vi "AuthAtServer.vi"(8 "password":string, 9 "login":string, 10 "Port":u32, 11 "Adress":string) -> (0 "MulticastAdress":string, 1 "AuthKey":string, 3 "error out":errorcluster)   [LabVIEW 2016]
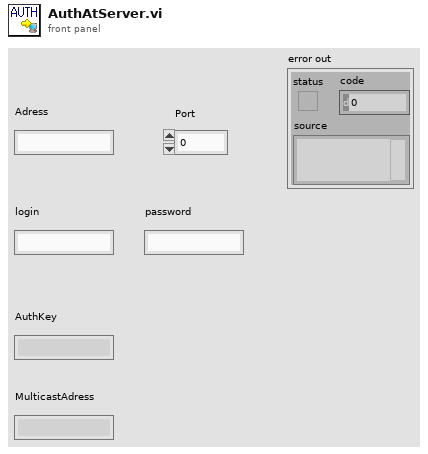
[diagram p1: front panel]
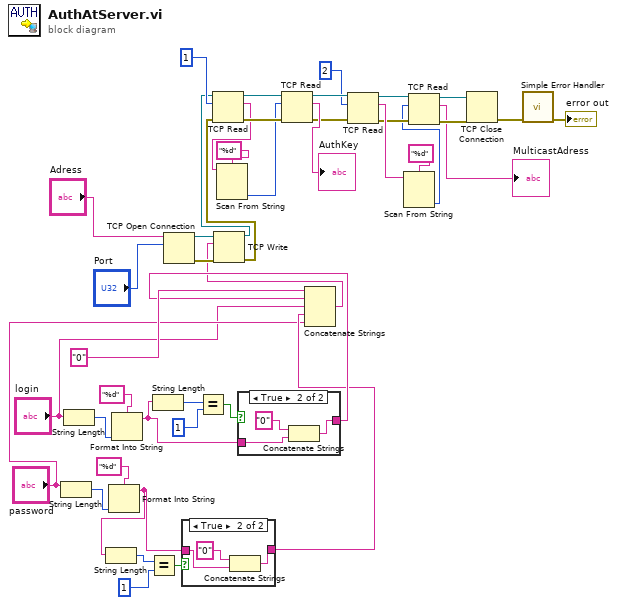
[diagram p0: block diagram]
diagram:
  n1 = String Length(string="password") -> (length=w39:i32)
  n2 = String Length(string="login") -> (length=w41:i32)
  n3 = Format Into String(format string="%d", w39) -> (resulting string=w32:string)  [unwired: 2 in, 1 out]
  n4 = String Length(string=w32) -> (length=w35:i32)
  n5 = Format Into String(format string="%d", w41) -> (resulting string=w28:string)  [unwired: 2 in, 1 out]
  n6 = Equal?(x=w35, y=1) -> (x = y?=w33:bool)
  n7 = String Length(string=w28) -> (length=w31:i32)
  n8 = TCP Open Connection(address="Adress", remote port or service name="Port") -> (connection ID=w42:refnum<k5>, error out=w43:errorcluster)  [unwired: 3 in]
  n9 = case shown="True" w33 {
    tunnel: w32 -> [w45 w47]
    tunnel: [w45 w46] -> w4
    frame False {
    }
    frame True {
      n10 = Concatenate Strings("0", w47) -> (w46:string)
    }
  }
  n11 = Equal?(x=w31, y=1) -> (x = y?=w29:bool)
  n12 = case shown="True" w29 {
    tunnel: w28 -> [w49 w51]
    tunnel: [w49 w50] -> w7
    frame False {
    }
    frame True {
      n13 = Concatenate Strings("0", w51) -> (w50:string)
    }
  }
  n14 = Concatenate Strings("0", w7, "login", w4, "password") -> (w1:string)
  n15 = TCP Write(connection ID=w42, data in=w1, error in (no error)=w43) -> (connection ID out=w6:refnum<k5>, error out=w5:errorcluster)  [unwired: 1 in, 1 out]
  n16 = TCP Read(connection ID=w6, bytes to read=1, error in (no error)=w5) -> (connection ID out=w26:refnum<k5>, data out=w25:string, error out=w27:errorcluster)  [unwired: 2 in]
  n17 = Scan From String(format string="%d", input string=w25) -> (output 1=w23:i32)  [unwired: 3 in, 3 out]
  n18 = TCP Read(connection ID=w26, bytes to read=w23, error in (no error)=w27) -> (connection ID out=w19:refnum<k5>, data out=→"AuthKey":string, error out=w18:errorcluster)  [unwired: 2 in]
  n19 = TCP Read(connection ID=w19, bytes to read=2, error in (no error)=w18) -> (connection ID out=w13:refnum<k5>, data out=w15:string, error out=w14:errorcluster)  [unwired: 2 in]
  n20 = Scan From String(format string="%d", input string=w15) -> (output 1=w12:i32)  [unwired: 3 in, 3 out]
  n21 = TCP Read(connection ID=w13, bytes to read=w12, error in (no error)=w14) -> (connection ID out=w11:refnum<k5>, data out=→"MulticastAdress":string, error out=w10:errorcluster)  [unwired: 2 in]
  n22 = TCP Close Connection(connection ID=w11, error in (no error)=w10) -> (error out=w37:errorcluster)  [unwired: 1 in, 1 out]
  n23 = call <vilib>:"Simple Error Handler.vi"("error in (no error)"=w37) -> ("error out"=→"error out":errorcluster)  [unwired: 4 in, 4 out]
